vi "CreateNew_IncludeItem.vi"(11 "Wizard":T1) -> (3 "Include me":bool)   [LabVIEW 2020, in "FlexWorker_Provider.lvlib"]
uses:
  FlexWorker_Provider.lvlib
  <resource>/Framework/Providers/API/ItemRef.ctl
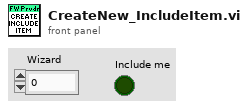
[diagram p1: front panel]
types:
  T1 = typedef "ItemRef.ctl" = u64
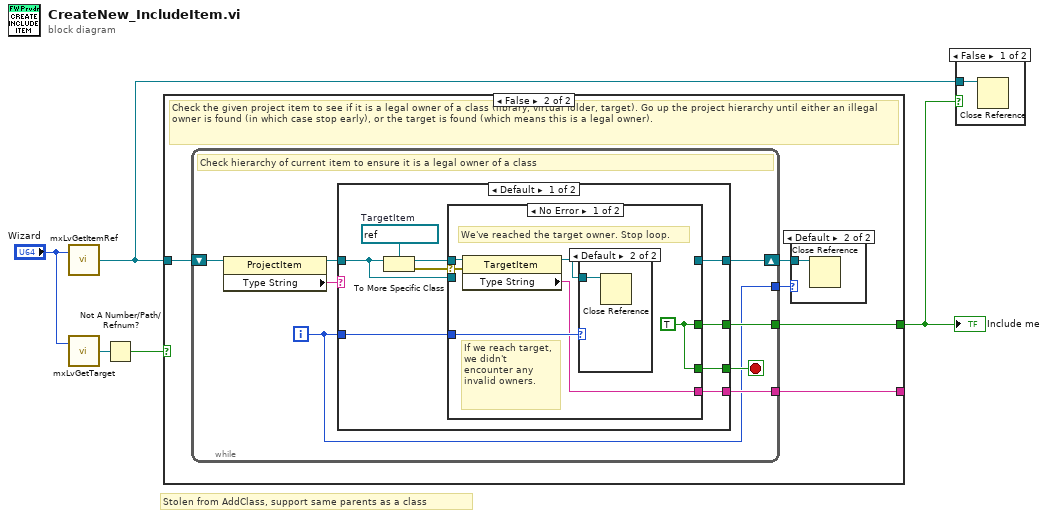
[diagram p0: block diagram]
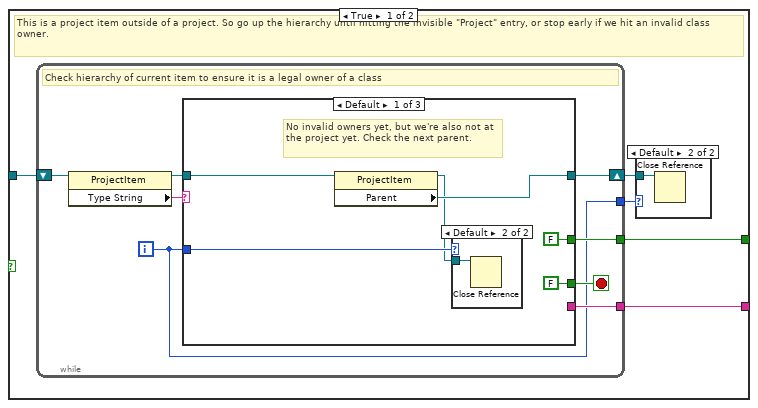
[diagram p3: hidden frame]
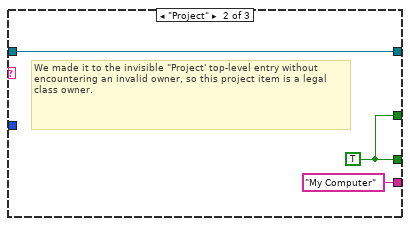
[diagram p6: hidden frame]
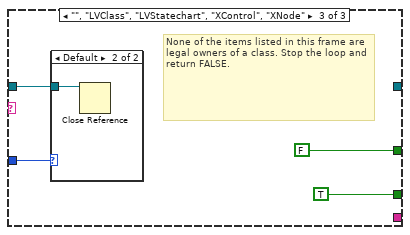
[diagram p7: hidden frame]
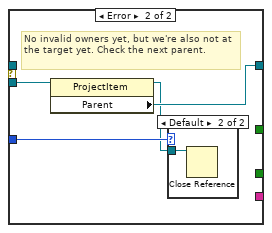
[diagram p11: hidden frame]
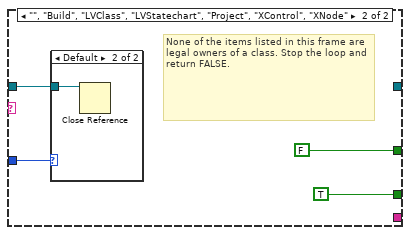
[diagram p13: hidden frame]
diagram:
  # "Stolen from AddClass, support same parents as a class"
  n1 = call <resource>:"mxLvGetItemRef.vi"("Item"="Wizard") -> ("Item Refnum"=w1:refnum<vi>)  [unwired: 1 in, 2 out]
  n2 = call <resource>:"mxLvGetTarget.vi"("Item"="Wizard") -> ("Target"=w4:refnum<vi>)  [unwired: 1 in, 2 out]
  n3 = Not A Number/Path/Refnum?(number/path/refnum=w4) -> (NaN/Path/Refnum?=w3:bool)
  n4 = case shown="False" w3 {
    tunnel: [w10 w39] -> w2
    tunnel: [w8 w37] -> _
    tunnel: w1 -> [w7 w36]
    frame True {
      # "This is a project item outside of a project. So go up the hierarchy until hitting the invisible \"Project\" entry, or stop early if we hit an invalid class owner."
      n5 = while {
        shift-right: [w14] -> w9
        shift-left: w7 -> [w19]
        tunnel: [w16] -> w10
        tunnel: [w13] -> w8
        tunnel: [w12] -> w6
        i -> [w12]
        stop <- w17 stop-if-true
        # "Check hierarchy of current item to ensure it is a legal owner of a class"
        n6 = property class="ProjectItem"(reference=w19) -> (reference out=w15:refnum<vi>, "Type String"=w18:string)  [unwired: 1 in, 1 out]
        n7 = case shown="Default" w18 {
          tunnel: [FALSE w29 TRUE] -> w17
          tunnel: [FALSE w29 FALSE] -> w16
          tunnel: w15 -> [w25 w27 w30]
          tunnel: [w24 w27 _] -> w14
          tunnel: w12 -> [w23 _ w31]
          tunnel: [_ "My Computer" ("Type String") _] -> w13
          frame Default {
            # "No invalid owners yet, but we're also not at the project yet. Check the next parent."
            n8 = property class="ProjectItem"(reference=w25) -> (reference out=w22:refnum<vi>, "Parent"=w24:refnum<vi>)  [unwired: 1 in, 1 out]
            n9 = case shown="Default" w23 {
              tunnel: w22 -> [_ w26]
              frame 0 {
              }
              frame Default {
                n10 = Close Reference(reference=w26) -> ()  [unwired: 1 in, 1 out]
              }
            }
          }
          frame "Project" {
            w29 = TRUE
            # "We made it to the invisible \"Project' top-level entry without encountering an invalid owner, so this project item is a legal class owner."
          }
          frame "", "LVClass", "LVStatechart", "XControl", "XNode" {
            # "None of the items listed in this frame are legal owners of a class. Stop the loop and return FALSE."
            n11 = case shown="Default" w31 {
              tunnel: w30 -> [_ w34]
              frame 0 {
              }
              frame Default {
                n12 = Close Reference(reference=w34) -> ()  [unwired: 1 in, 1 out]
              }
            }
          }
        }
      }
      n13 = case shown="Default" w6 {
        tunnel: w9 -> [_ w11]
        frame 0 {
        }
        frame Default {
          n14 = Close Reference(reference=w11) -> ()  [unwired: 1 in, 1 out]
        }
      }
    }
    frame False {
      # "Check the given project item to see if it is a legal owner of a class (library, virtual folder, target). Go up the project hierarchy until either an illegal owner is found (in which case stop early), or the target is found (which means this is a legal owner)."
      n15 = while {
        shift-right: [w43] -> w38
        shift-left: w36 -> [w48]
        tunnel: [w45] -> w39
        tunnel: [w42] -> w37
        tunnel: [w41] -> w35
        i -> [w41]
        stop <- w46 stop-if-true
        # "Check hierarchy of current item to ensure it is a legal owner of a class"
        n16 = property class="ProjectItem"(reference=w48) -> (reference out=w44:refnum<vi>, "Type String"=w47:string)  [unwired: 1 in, 1 out]
        n17 = case shown="Default" w47 {
          tunnel: [w54 TRUE] -> w46
          tunnel: [w55 FALSE] -> w45
          tunnel: w44 -> [w53 w70]
          tunnel: [w52 _] -> w43
          tunnel: w41 -> [w51 w71]
          tunnel: [w49 _] -> w42
          frame Default {
            w57 = refnum<vi> refnum  # TargetItem
            n18 = To More Specific Class(target class=w57, reference=w53) -> (specific class reference=w50:refnum<vi>, error out=w56:errorcluster)  [unwired: 1 in]
            n19 = case shown="No Error" w56 {
              selector: w56 -> [w60 _]
              tunnel: [w63 _] -> w55
              tunnel: [w63 _] -> w54
              tunnel: w53 -> [_ w68]
              tunnel: [_ w67] -> w52
              tunnel: w51 -> [w62 w66]
              tunnel: w50 -> [w61 _]
              tunnel: [w58 _] -> w49
              frame No Error {
                w63 = TRUE
                # "If we reach target, we didn't encounter any invalid owners."
                # "We've reached the target owner. Stop loop."
                n20 = property class="TargetItem"(reference=w61, error in=w60) -> (reference out=w59:refnum<vi>, "Type String"=w58:string)  [unwired: 1 out]
                n21 = case shown="Default" w62 {
                  tunnel: w59 -> [_ w64]
                  frame 0 {
                  }
                  frame Default {
                    n22 = Close Reference(reference=w64) -> ()  [unwired: 1 in, 1 out]
                  }
                }
              }
              frame Error {
                # "No invalid owners yet, but we're also not at the target yet. Check the next parent."
                n23 = property class="ProjectItem"(reference=w68) -> (reference out=w65:refnum<vi>, "Parent"=w67:refnum<vi>)  [unwired: 1 in, 1 out]
                n24 = case shown="Default" w66 {
                  tunnel: w65 -> [_ w69]
                  frame 0 {
                  }
                  frame Default {
                    n25 = Close Reference(reference=w69) -> ()  [unwired: 1 in, 1 out]
                  }
                }
              }
            }
          }
          frame "", "Build", "LVClass", "LVStatechart", "Project", "XControl", "XNode" {
            # "None of the items listed in this frame are legal owners of a class. Stop the loop and return FALSE."
            n26 = case shown="Default" w71 {
              tunnel: w70 -> [_ w74]
              frame 0 {
              }
              frame Default {
                n27 = Close Reference(reference=w74) -> ()  [unwired: 1 in, 1 out]
              }
            }
          }
        }
      }
      n28 = case shown="Default" w35 {
        tunnel: w38 -> [_ w40]
        frame 0 {
        }
        frame Default {
          n29 = Close Reference(reference=w40) -> ()  [unwired: 1 in, 1 out]
        }
      }
    }
  }
  "Include me" <- w2
  n30 = case shown="False" w2 {
    tunnel: w1 -> [w75 _]
    frame False {
      n31 = Close Reference(reference=w75) -> ()  [unwired: 1 in, 1 out]
    }
    frame True {
    }
  }
